vi "Teleop.vi"(10 "Match Info":T1={"Autonomous Elapsed Seconds"=0.0, "TeleOp Elapsed Seconds"=0.0, "Disabled Elapsed Seconds"=0.0, "Visited Autonomous"=FALSE, "Visited TeleOp"=FALSE, "Visited Disabled"=FALSE, "Autonomous Settings"={"Autonomous Style"=enum."Independent", "VI Refnum"=refnum}}, 11 "Call Context":T2) -> ()   [LabVIEW 2020]
doc: "This VI is called for each TeleOp packet received from the DS where the robot is not disabled. It is often used to read from the joysticks and update I/O or to update setpoints for timed control loops. It should complete and return within 20 milliseconds or it may miss DS packets."
uses:
  <vilib>/Rock Robotics/WPI/DriverStation/WPI_DriverStationDerivedRobotMode.ctl
  <vilib>/Rock Robotics/WPI/DriverStation/WPI_DriverStationMatch Info.ctl
  <vilib>/Rock Robotics/WPI/RobotDrive/WPI_RobotDriveMecanumDrive_Cartesian.vi
  <vilib>/addons/control/pid/NI_PID_pid.lvlib
  <vilib>/addons/control/pid/pid.llb/PID (DBL).vi
  Control 4.ctl
panel:
  out "Sample Slider 0":dbl format="%#_13g"
  out "Sample Boolean 1":bool=TRUE
  out "Sample Boolean 0":bool=TRUE
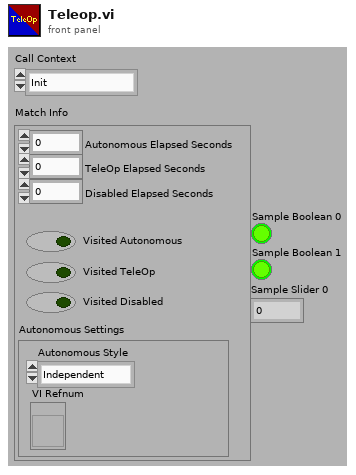
[diagram p1: front panel]
types:
  T1 = typedef "WPI_DriverStationMatch Info.ctl" = cluster{"Autonomous Elapsed Seconds":dbl, "TeleOp Elapsed Seconds":dbl, "Disabled Elapsed Seconds":dbl, "Visited Autonomous":bool, "Visited TeleOp":bool, "Visited Disabled":bool, "Autonomous Settings":cluster{"Autonomous Style":enum16{"Iterative", "Independent"}, "VI Refnum":refnum<vi>}}
  T2 = typedef "WPI_DriverStationDerivedRobotMode.ctl" = enum16{"Init", "Execute", "Stop"}
  T3 = typedef "Control 4.ctl" = enum16{"Dev0", "Dev1", "Dev2", "Dev3"}
  T4 = typedef "WPI_JoystickDevRef.ctl" = cluster{"Device":T5}
  T5 = typedef "WPI_JoystickDeviceEnum.ctl" = enum16{"USB 0", "USB 1", "USB 2", "USB 3", "USB 4", "USB 5"}
  T6 = typedef "WPI_RobotDriveDevRef.ctl" = cluster{"DevStatus":errorcluster, "Motors[]":T7[], "Square Inputs":bool, "Max Output":dbl}
  T7 = typedef "WPI_MotorControlDeviceRef.ctl" = cluster{"DeviceStatus":errorcluster, "Type":T8, "PWM":cluster{"PWM Channel":T9, "DeadBand":T10}, "CAN":cluster{"Device Number":u8, "SetOutput VI Ref":variant, "GetOutput VI Ref":variant, "Enable VI Ref":variant, "Disable VI Ref":variant, "Data":variant}, "Invert":bool, "DIO PWM":cluster{"PWM \"Enable\" Channel":T9, "DIOChannel":T11, "PWM Rate":dbl}}
  T8 = typedef "WPI_MotorControlType.ctl" = enum16{"PWM", "CAN", "DIO PWM"}
  T9 = typedef "FPGA_DIOPWMChannel.ctl" = enum8{"PWM 0", "PWM 1", "PWM 2", "PWM 3", "PWM 4", "PWM 5", "PWM 6", "PWM 7", "PWM 8", "PWM 9", "PWM MXP 0", "PWM MXP 1", "PWM MXP 2", "PWM MXP 3", "PWM MXP 4", "PWM MXP 5", "PWM MXP 6", "PWM MXP 7", "PWM MXP 8", "PWM MXP 9", "Invalid"}
  T10 = typedef "WPI_PWMDeadband.ctl" = cluster{"Name":string, "maxPositivePwm":i32, "minPositivePwm":i32, "centerPwm":i32, "maxNegativePwm":i32, "minNegativePwm":i32, "angularRange":u16}
  T11 = typedef "FPGA_DIOChannel.ctl" = enum8{"DIO 0", "DIO 1", "DIO 2", "DIO 3", "DIO 4", "DIO 5", "DIO 6", "DIO 7", "DIO 8", "DIO 9", "DIO MXP 0", "DIO MXP 1", "DIO MXP 2", "DIO MXP 3", "DIO MXP 4", "DIO MXP 5", "DIO MXP 6", "DIO MXP 7", "DIO MXP 8", "DIO MXP 9", "DIO MXP 10", "DIO MXP 11", "DIO MXP 12", "DIO MXP 13", "DIO MXP 14", "DIO MXP 15", "SPI Port CS1", "SPI Port CS2", "SPI Port CS3", "SPI Port MISO", "SPI Port MOSI", "Invalid"}
  T12 = cluster{"Yaw":dbl, "Roll":dbl, "Pitch":dbl, "Heading":dbl, "Fused Heading":dbl}
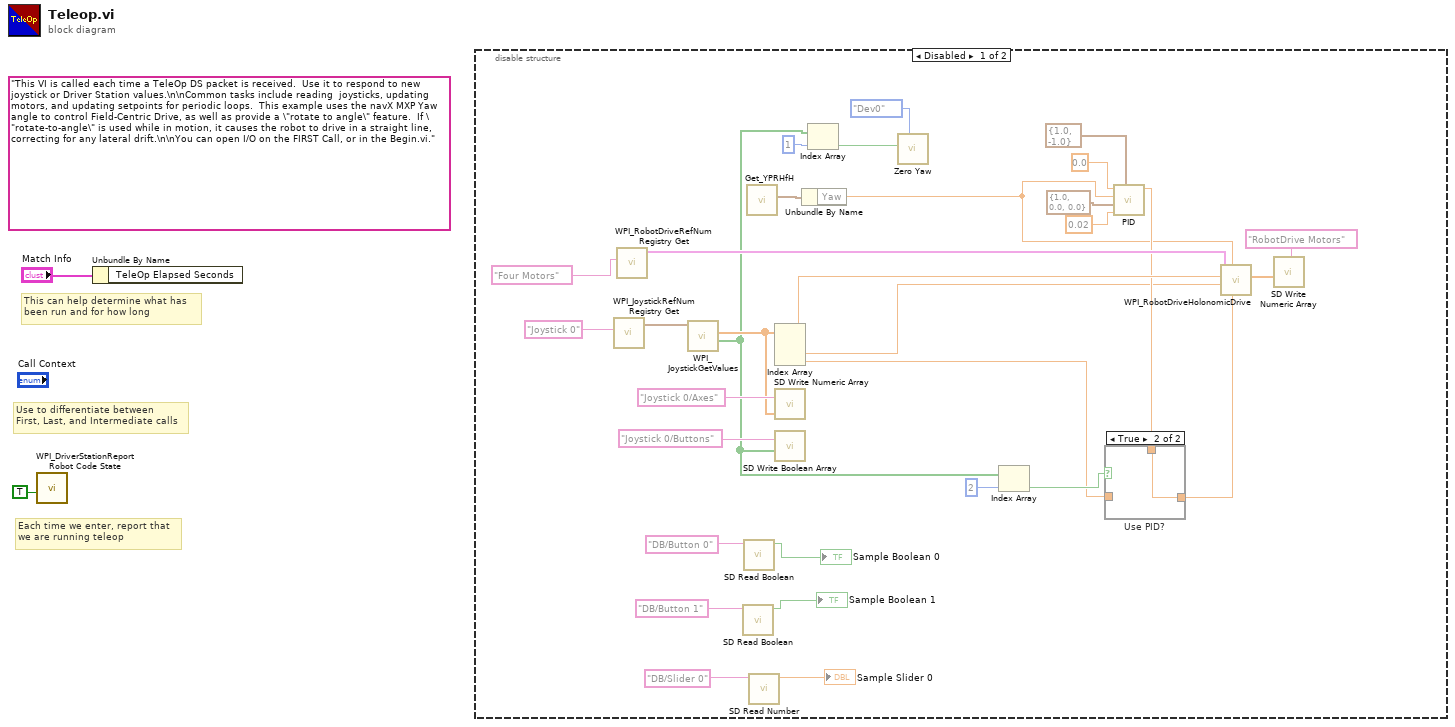
[diagram p0: block diagram]
diagram:
  (unwired) "This VI is called each time a TeleOp DS packet is received.  Use it to respond to new joystick or Driver Station values.\n\nCommon tasks include reading  joysticks, updating motors, and updating setpoints for periodic loops.  This example uses the navX MXP Yaw angle to control Field-Centric Drive, as well as provide a \"rotate to angle\" feature.  If \"rotate-to-angle\" is used while in motion, it causes the robot to drive in a straight line, correcting for any lateral drift.\n\nYou can open I/O on the FIRST Call, or in the Begin.vi."
  # "This can help determine what has\nbeen run and for how long"
  # "Use to differentiate between\nFirst, Last, and Intermediate calls"
  # "Each time we enter, report that\nwe are running teleop"
  n1 = call <vilib>:"WPI_DriverStationReport Robot Code State.vi"("TeleOp"=TRUE ("Autonomous")) -> ()  [unwired: 10 in, 1 out]
  n2 = Unbundle By Name("Match Info") -> ()  [unwired: 1 out]
  n3 = disable-structure shown="Disabled" {
    frame Disabled {
      n4 = call <vilib>:"WPI_JoystickRefNum Registry Get.vi"("refnum name"="Joystick 0") -> ("JoystickDevRef"=w34:T4)  [unwired: 9 in, 1 out]
      n5 = call <vilib>:"WPI_RobotDriveRefNum Registry Get.vi"("refnum name"="Four Motors") -> ("RobotDriveDevRef"=w30:T6)  [unwired: 9 in, 1 out]
      n6 = call <vilib>:"WPI_JoystickGetValues.vi"("JoystickDevRef"=w34) -> ("Buttons"=w6:bool[], "Axes"=w8:dbl[])  [unwired: 6 in, 3 out]
      n7 = call <vilib>:"SD Read Boolean.vi"("Name"="DB/Button 1") -> ("Boolean"=→"Sample Boolean 1":bool)  [unwired: 8 in, 2 out]
      n8 = call <vilib>:"SD Read Boolean.vi"("Name"="DB/Button 0") -> ("Boolean"=→"Sample Boolean 0":bool)  [unwired: 8 in, 2 out]
      n9 = call <vilib>:"Get_YPRHfH.vi"() -> ("YRPHfH"=w17:T12)  [unwired: 11 in]
      n10 = call <vilib>:"SD Read Number.vi"("Name"="DB/Slider 0") -> ("Numeric"=→"Sample Slider 0":dbl)  [unwired: 8 in, 2 out]
      n11 = Index Array(array=w8) -> (element #1=w29:dbl, element #2=w3:dbl, element #3=w25:dbl)  [unwired: 3 in]
      n12 = call <vilib>:"SD Write Numeric Array.vi"("Numeric Array"=w8, "Name"="Joystick 0/Axes") -> ()  [unwired: 8 in, 2 out]
      n13 = call <vilib>:"SD Write Boolean Array.vi"("Boolean Array"=w6, "Name"="Joystick 0/Buttons") -> ()  [unwired: 8 in, 2 out]
      n14 = Unbundle By Name(w17) -> ("Yaw"=w18:dbl)
      n15 = Index Array(array=w6, index=1) -> (element=w28:bool)
      n16 = call <vilib>:"Zero Yaw.vi"("Device Number"=Control_4."Dev0", "Zero"=w28) -> ()  [unwired: 10 in]
      n17 = Index Array(array=w6, index=2) -> (element=w26:bool)
      n18 = call-poly <vilib>:"PID.vi"("output range"=cluster{"Numeric 2":dbl, "Numeric 3":dbl} {"Numeric 2"=1.0, "Numeric 3"=-1.0}, "dt (s)"=0.02, "PID gains"=cluster{"Numeric 2":dbl, "Numeric 3":dbl, dbl} {"Numeric 2"=1.0, "Numeric 3"=0.0, 0.0}, "process variable"=w18, "setpoint"=0.0) -> ("output"=w23:dbl)  [unwired: 5 in, 1 out]
      n19 = case "Use PID?" shown="True" w26 {
        tunnel: w25 -> [w35 _]
        tunnel: [w35 w36] -> w24
        tunnel: w23 -> [_ w36]
        frame False {
        }
        frame True {
        }
      }
      n20 = call-poly <vilib>:"WPI_RobotDriveHolonomicDrive.vi"("Rotation"=w24, "Gyro Angle"=w18, "Y"=w3, "X"=w29, "RobotDriveDevRef"=w30) -> ("Motor Values"=w4:dbl[])  [unwired: 4 in, 2 out]
      n21 = call <vilib>:"SD Write Numeric Array.vi"("Numeric Array"=w4, "Name"="RobotDrive Motors") -> ()  [unwired: 8 in, 2 out]
    }
    frame Enabled {
    }
  }
